vi "E-Series Reader tester.vi"() -> ()   [LabVIEW 2018, in "E-Series Reader.lvlib"]
uses:
  E-Series Reader.lvlib
  series data--control.ctl
panel:
  in  "E Series File Names":string[](array[string])=["E3 Series.csv", "E6 Series.csv", "E12 Series.csv", "E24 Series.csv", "E48 Series.csv", "E96 Series.csv", "E192 Series.csv"]
  out "Series Data":T1
  # "Tester for \nCSV Series Reader VI"
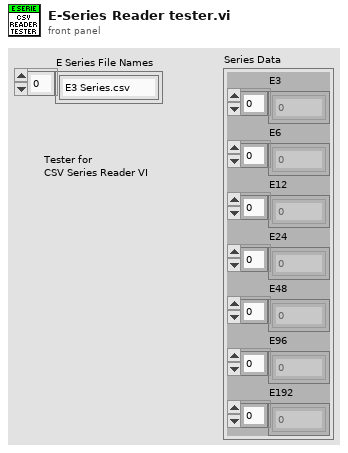
[diagram p1: front panel]
types:
  T1 = typedef "E-Series Reader.lvlib/series data--control.ctl" = cluster{"E3":u16[], "E6":u16[], "E12":u16[], "E24":u16[], "E48":u16[], "E96":u16[], "E192":u16[]}
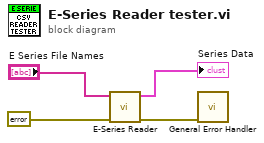
[diagram p0: block diagram]
diagram:
  n1 = call "E-Series Reader.vi"("error in"=errorcluster {"status"=FALSE, "code"=0, "source"=""}, "E Series File Names"="E Series File Names") -> ("error out"=w1:errorcluster, "Series Data"=→"Series Data":T1)  [unwired: 8 in]
  n2 = call <vilib>:"General Error Handler.vi"("error in (no error)"=w1) -> ()  [unwired: 10 in, 5 out]
